vi "Read Has Value.vi"(8 "error in (no error)":errorcluster, 11 "Proto Type Common in":refnum<class "Proto Type Data Base.lvclass">) -> (0 "error out":errorcluster, 2 "Value Set":bool, 3 "Proto Type Common out":refnum<class "Proto Type Data Base.lvclass">)   [LabVIEW 2020, in "Protobuf RAW.lvlib" / "Proto Type Data Base.lvclass"]
uses:
  Proto Type Data Base.lvclass
  Proto Type Data Base.lvclass/Proto Type Data Base.ctl
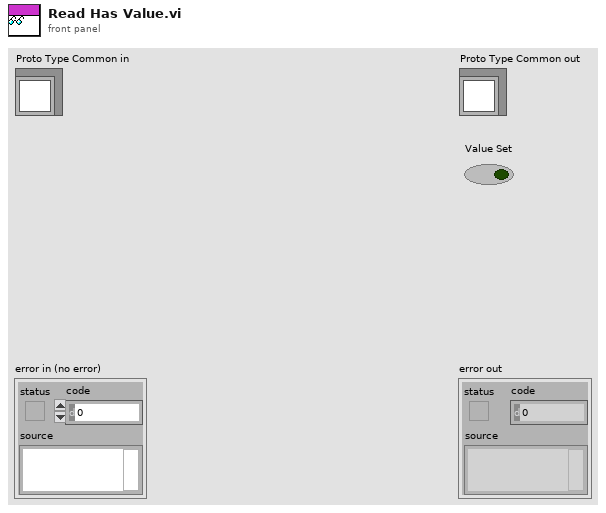
[diagram p1: front panel]
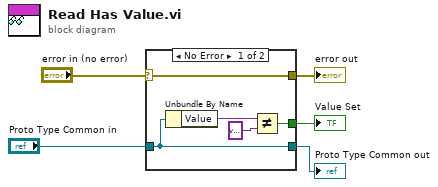
[diagram p0: block diagram]
diagram:
  n1 = case shown="No Error" "error in (no error)" {
    selector: "error in (no error)" -> [w10 w11]
    tunnel: [w10 w11] -> w4
    tunnel: [w9 w12] -> w2
    tunnel: "Proto Type Common in" -> [w9 w12]
    tunnel: [w6 _] -> w1
    frame No Error {
      n2 = Unbundle By Name(w9) -> ("Value"=w7:variant)
      n3 = Not Equal?(x=w7, y=variant) -> (x != y?=w6:bool)
    }
    frame Error {
    }
  }
  "error out" <- w4
  "Proto Type Common out" <- w2
  "Value Set" <- w1
